vi "Read Value Class.vi"(8 "error in (no error)":errorcluster, 11 "abs_Type Leaf in":refnum<class "abs_Type Leaf.lvclass">) -> (0 "error out":errorcluster, 2 "Abs_Type.lvclass":refnum<class "Abs_Type.lvclass">, 3 "abs_Type Leaf out":refnum<class "abs_Type Leaf.lvclass">)   [LabVIEW 2021, in "BT.lvlib" / "abs_Type Leaf.lvclass"]
uses:
  abs_Type Leaf.lvclass
  <vilib>/TSA/Abstract Data Classes/Abs_Types/Type/Abs_Type.lvclass
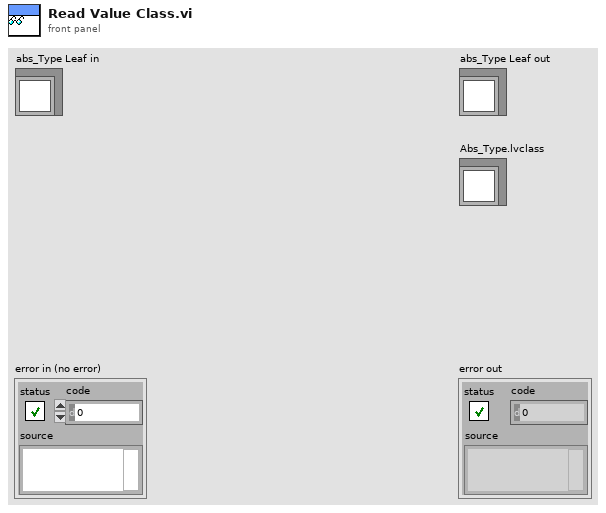
[diagram p1: front panel]
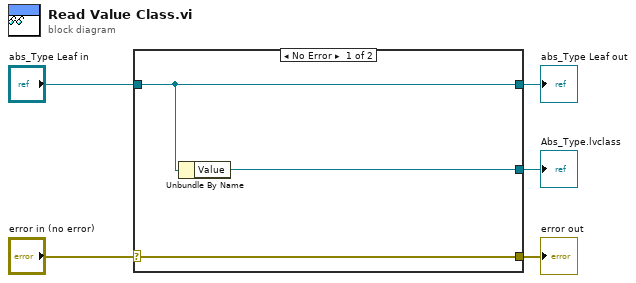
[diagram p0: block diagram]
diagram:
  n1 = case shown="No Error" "error in (no error)" {
    selector: "error in (no error)" -> [w8 w9]
    tunnel: [w8 w9] -> w4
    tunnel: [w7 w10] -> w2
    tunnel: "abs_Type Leaf in" -> [w7 w10]
    tunnel: [w6 _] -> w1
    frame No Error {
      n2 = Unbundle By Name(w7) -> ("Value"=w6:refnum<class "Abs_Type.lvclass">)
    }
    frame Error {
    }
  }
  "error out" <- w4
  "abs_Type Leaf out" <- w2
  "Abs_Type.lvclass" <- w1
